vi "cmd_move.vi"(8 "error in (no error)":errorcluster, 11 "JSON":string) -> (0 "error out":errorcluster)   [LabVIEW 2021]
doc: "Change output target\n\n You can specify the output channel and value.\n \n :param ch: Specifies the output channel\n :param val: Specifies the output values"
uses:
  fpga/fpga_dtype_scan_config.ctl
  fpga/fpga_dtype_sgl_8ch.ctl
  fpga/fpga_dtype_index.ctl
panel:
  in  "args":cluster{"ch":i32, "val":sgl}
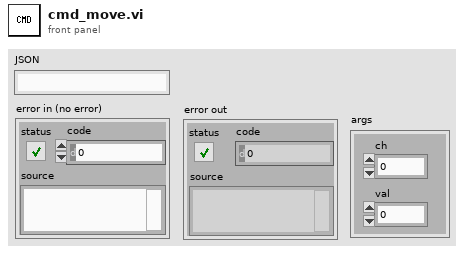
[diagram p1: front panel]
types:
  T1 = typedef "fpga_dtype_index.ctl" = cluster{"page":i16, "2nd":i16, "1st":i16}
  T2 = typedef "fpga_dtype_scan_config.ctl" = cluster{"data points":i16, "average counts":i16, "delta per point":T3, "bidirectional scan":bool, "auto reversal":bool}
  T3 = typedef "fpga_dtype_sgl_8ch.ctl" = cluster{"ch 0":sgl, "ch 1":sgl, "ch 2":sgl, "ch 3":sgl, "ch 4":sgl, "ch 5":sgl, "ch 6":sgl, "ch 7":sgl}
  T4 = cluster{"target[0]":sgl, "target[1]":sgl, "target[2]":sgl, "target[3]":sgl, "target[4]":sgl, "target[5]":sgl, "target[6]":sgl, "target[7]":sgl}
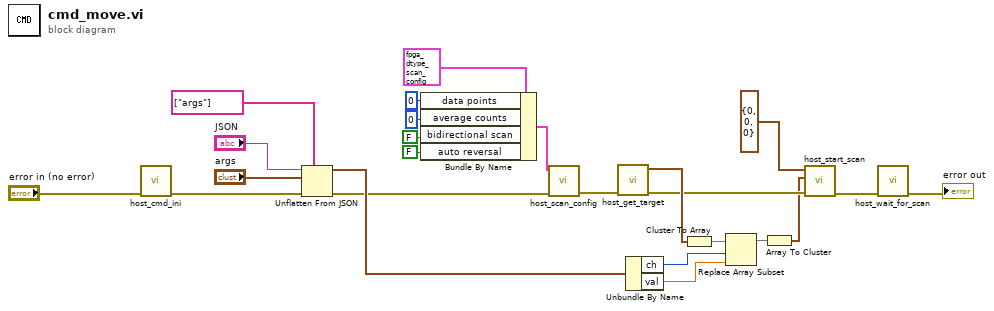
[diagram p0: block diagram]
diagram:
  n1 = call "host_cmd_ini.vi"("error in (no error)"="error in (no error)") -> ("error out"=w4:errorcluster)  [unwired: 10 in]
  n2 = Unflatten From JSON(path=string[] ["args"], JSON string="JSON", type and defaults="args", error in (no error)=w4) -> (value=w21:cluster{"ch":i32, "val":sgl}, error out=w20:errorcluster)  [unwired: 3 in]
  n3 = Bundle By Name(cluster=T2 {"data points"=0, "average counts"=0, "delta per point"={"ch 0"=0.0, "ch 1"=0.0, "ch 2"=0.0, "ch 3"=0.0, "ch 4"=0.0, "ch 5"=0.0, "ch 6"=0.0, "ch 7"=0.0}, "bidirectional scan"=FALSE, "auto reversal"=FALSE} ("scan config"), "data points"=i16 0, "average counts"=i16 0, "bidirectional scan"=FALSE, "auto reversal"=FALSE) -> (w16:T2)
  n4 = call "host_scan_config.vi"("error in"=w20, "scan config"=w16) -> ("error out"=w13:errorcluster)  [unwired: 9 in]
  n5 = call "host_get_target.vi"("error in"=w13) -> ("error out"=w8:errorcluster, "target"=w12:T3)  [unwired: 9 in]
  n6 = Unbundle By Name(w21) -> ("ch"=w10:i32, "val"=w9:sgl)
  n7 = Cluster To Array(cluster=w12) -> (array=w11:sgl[])
  n8 = Replace Array Subset(array=w11, new element=w9, index=w10) -> (w6:sgl[])
  n9 = Array To Cluster(array=w6) -> (cluster=w5:T4)
  n10 = call "host_start_scan.vi"("error in"=w8, "initial positions"=w5, "index offset"=T1 {"page"=0, "2nd"=0, "1st"=0}) -> ("error out"=w2:errorcluster)  [unwired: 6 in, 2 out]
  n11 = call "host_wait_for_scan.vi"("error in (no error)"=w2) -> ("error out"=→"error out":errorcluster)  [unwired: 10 in]
